vi "lab2.vi"() -> ()   [LabVIEW 2023]
uses:
  Control 1.ctl
panel:
  out "?":bool
  in  "Limitare":T1 caption="Limits"
  in  "MAX":dbl(slide) scale=0.0..10.0
  in  "MIN":dbl(slide) scale=0.0..10.0
  out "?":dbl(slide) scale=0.0..10.0
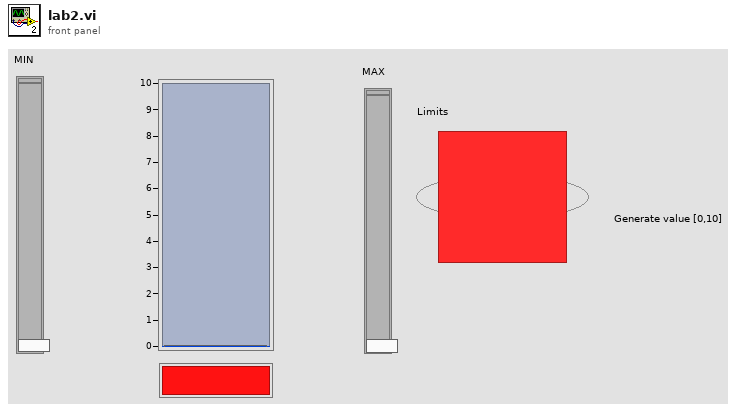
[diagram p1: front panel]
types:
  T1 = typedef "Control 1.ctl" = bool
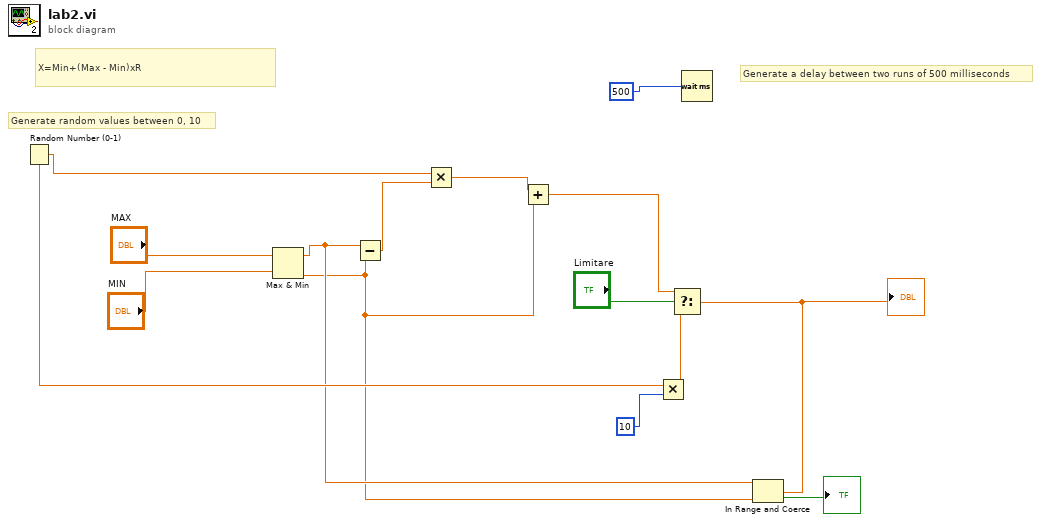
[diagram p0: block diagram]
diagram:
  # "Generate random values between 0, 10"
  # "X=Min+(Max - Min)xR"
  # "Generate a delay between two runs of 500 milliseconds"
  n1 = Random Number (0-1)() -> (number: 0 to 1=w10:dbl)
  n2 = Max & Min(x="MAX", y="MIN") -> (max(x,y)=w8:dbl, min(x,y)=w7:dbl)
  n3 = Subtract(x=w8, y=w7) -> (x-y=w12:dbl)
  n4 = Multiply(x=w10, y=w12) -> (x*y=w11:dbl)
  n5 = Add(x=w11, y=w7) -> (x+y=w5:dbl)
  n6 = Multiply(x=w10, y=10) -> (x*y=w4:dbl)
  n7 = Select(t=w5, s="Limitare", f=w4) -> (s? t:f=w3:dbl)
  "?" <- w3
  n8 = Wait (ms)(milliseconds to wait=500) -> ()  [unwired: 1 out]
  n9 = In Range and Coerce(upper limit=w8, x=w3, lower limit=w7) -> (In Range?=→"?":bool)  [unwired: 1 out]
